vi "Panel Init.vi"(8 "error in (no error)":errorcluster, 11 "PanelManager in":refnum<class "PanelManager.lvclass">) -> (0 "error out":errorcluster, 3 "PanelManager out":refnum<class "PanelManager.lvclass">)   [LabVIEW 2015, in "PanelManager.lvclass"]
uses:
  PanelManager.lvclass
  PanelManager.lvclass/PanelManager.ctl
  Type Definition/g_Panel_Data.ctl
  <vilib>/ActorFramework/Message Enqueuer/Message Enqueuer.lvclass
  Controller/BackStage.lvclass
  Controller/BackStage.lvclass/BackStage.ctl
  <vilib>/ActorFramework/Actor/Actor.lvclass
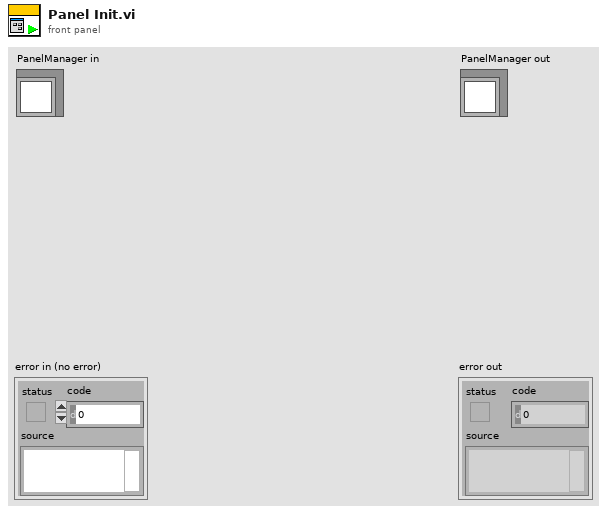
[diagram p1: front panel]
types:
  T1 = typedef "g_Panel_Data.ctl" = cluster{"BlackStage Queue":refnum<class "Message Enqueuer.lvclass">, "UI Dict":variant}
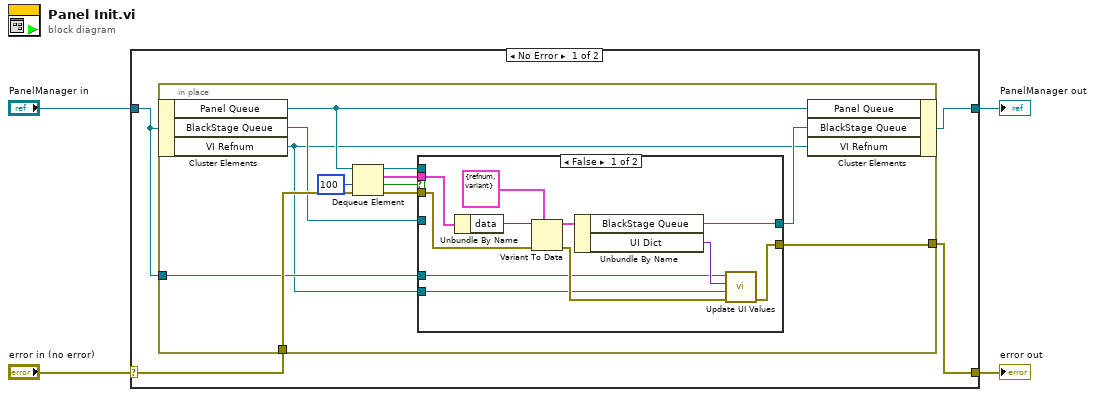
[diagram p0: block diagram]
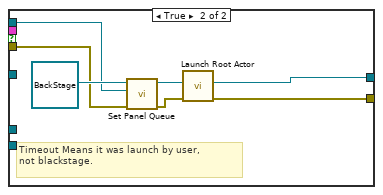
[diagram p2: hidden frame]
diagram:
  n1 = case shown="No Error" "error in (no error)" {
    selector: "error in (no error)" -> [w8 w40]
    tunnel: [w7 w40] -> w3
    tunnel: [w5 w39] -> w1
    tunnel: "PanelManager in" -> [w6 w39]
    frame No Error {
      n2 = in-place {
        in-place-border: w8 -> [w20]
        in-place-border: [w11] -> w7
        in-place-border: w6 -> [w10]
        n3 = in-place-cluster #1(w6) -> ("Panel Queue"=w14:refnum<queue>, "BlackStage Queue"=w12:refnum<class "Message Enqueuer.lvclass">, "VI Refnum"=w9:refnum<vi>)
        n4 = Dequeue Element(queue=w14, timeout in ms (-1)=100, error in (no error)=w20) -> (queue out=w17:refnum<queue>, element=w15:cluster{"cmd":string, "data":variant}, timed out?=w18:bool, error out=w16:errorcluster)
        n5 = case shown="False" w18 {
          tunnel: w17 -> [_ w35]
          tunnel: w16 -> [w28 w33]
          tunnel: w15 -> [w31 _]
          tunnel: [w26 w38] -> w13
          tunnel: w12 -> [_ _]
          tunnel: [w21 w37] -> w11
          tunnel: w10 -> [w22 _]
          tunnel: w9 -> [w23 _]
          frame False {
            n6 = Unbundle By Name(w31) -> ("data"=w30:variant)
            n7 = Variant To Data(error in=w28, type=T1 {"BlackStage Queue"=refnum, "UI Dict"=variant} ("g_panel Data"), Variant=w30) -> (data=w27:T1, error out=w24:errorcluster)
            n8 = Unbundle By Name(w27) -> ("BlackStage Queue"=w26:refnum<class "Message Enqueuer.lvclass">, "UI Dict"=w25:variant)
            n9 = call "Update UI Values.vi"("error in (no error)"=w24, "This VI"=w23, "Controls Value"=w25, "PanelManager in"=w22) -> ("error out"=w21:errorcluster)  [unwired: 6 in, 1 out]
          }
          frame True {
            # "Timeout Means it was launch by user, \nnot blackstage."
            n10 = call "Set Panel Queue.vi"("error in (no error)"=w33, "Panel Queue"=w35, "BackStage in"=refnum<class "BackStage.lvclass"> refnum ("BackStage.lvclass")) -> ("error out"=w32:errorcluster, "BackStage out"=w34:refnum<class "BackStage.lvclass">)  [unwired: 7 in]
            n11 = call <vilib>:"Launch Root Actor.vi"("error in (no error)"=w32, "Actor"=w34) -> ("error out"=w37:errorcluster, "Actor's Enqueuer"=w38:refnum<class "Message Enqueuer.lvclass">)  [unwired: 8 in]
          }
        }
        n12 = in-place-cluster #1("Panel Queue"=w14, "BlackStage Queue"=w13, "VI Refnum"=w9) -> (w5:refnum<class "PanelManager.lvclass">)
      }
    }
    frame Error {
    }
  }
  "error out" <- w3
  "PanelManager out" <- w1
